vi "Test Copy from Pixmap Greyscale.vi"(8 "error in (no error)":errorcluster, 11 "Test Case In":refnum<class "Image.lvclass">) -> (0 "error out":errorcluster, 3 "Test Case Out":refnum<class "Image.lvclass">)   [LabVIEW 2020, in "test.lvlib" / "Image.lvclass"]
uses:
  Image.lvclass
  C:/Program Files (x86)/National Instruments/LabVIEW 2020/vi.lib/Astemes/LUnit/Test Case.lvclass
  <vilib>/picture/picture.llb/imagedata.ctl
  <vilib>/Astemes/LUnit/Test Case.lvclass/Test Case.ctl
  2c93f62b-78d7-4b59-b27c-14bd701a5d71.vi
  8166983f-db3b-480f-a786-a958408166cb.vi
  03fde0f0-e029-4dad-9f9a-a95d25ce423a.vi
  3bb2986f-6074-4300-8ef6-a7ee1c3ba308.vi
  02fb1d00-84d2-4392-bb0c-78c1f80e642d.vi
  image/New Image (Greyscale).vi
  image/Copy Pixmap to Image (Greyscale with Mask Output).vi
  image/Copy Pixmap to Image (Greyscale Flatten Mask).vi
  7f5bb767-9dbf-47d9-8f44-5f4901e96d00.vi
  e6d5ae8e-bd70-4c65-a769-b7cfb03e80c7.vi
  d454bffa-6717-48ab-b8d5-b1f03345aa55.vi
  image/New Image (Greyscale).vi/6598b9e0-8a08-46f5-91fd-ca1b87217137.vi
  image/Copy Pixmap to Image (Greyscale with Mask Output).vi/3b7a14f1-ed28-461e-8305-e3c68bcd5d6e.vi
  image/Copy Pixmap to Image (Greyscale Flatten Mask).vi/f0818824-bd55-4656-87f2-fcc208e7cf24.vi
  <vilib>/Astemes/LUnit/Append Pass Result.vi
  <vilib>/Astemes/LUnit/Append Fail Result.vi
  <vilib>/Astemes/LUnit/Describe Comparison.vi
  7f5bb767-9dbf-47d9-8f44-5f4901e96d00.vi/9c5d11cd-9439-4240-a1ee-d9baace9c924.vi
  e6d5ae8e-bd70-4c65-a769-b7cfb03e80c7.vi/9c5d11cd-9439-4240-a1ee-d9baace9c924.vi
  d454bffa-6717-48ab-b8d5-b1f03345aa55.vi/9c5d11cd-9439-4240-a1ee-d9baace9c924.vi
  image/FixPixmap.vi
  <vilib>/Astemes/LUnit/Run In UI.vi
  image/Default8bitColourMap.vi
  <vilib>/Utility/error.llb/Clear Errors.vi
  <vilib>/Utility/colorconv.llb/Color to RGB.vi
  common/Module Path.vi
  <vilib>/Utility/error.llb/Error Cluster From Error Code.vi
  <vilib>/Astemes/LUnit/Describe Variant.vi
  image/image.lvlib
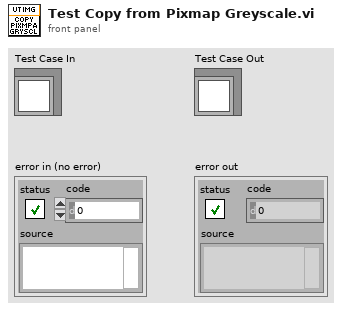
[diagram p1: front panel]
types:
  T1 = enum16{"8 Bit No Mask", "24 Bit No Mask", "32 Bit No Mask", "8 Bit Mask", "24 Bit Mask", "32 Bit Mask", "8 Pixels Wide Masked", "16 Pixels Wide Masked"}
  T2 = cluster{"left":i16, "top":i16, "right":i16, "bottom":i16}
  T3 = enum16{"8 Bit No Mask", "24 Bit No Mask", "32 Bit No Mask", "8 Bit Mask", "24 Bit Mask", "32 Bit Mask", "8 Pixels Wide Masked", "16 Pixels Wide Masked"}[]
  T4 = typedef "imagedata.ctl" = cluster{"image type":i32, "image depth":i32, "image":u8[], "mask":u8[], "colors":u32[], "Rectangle":cluster{"left":i16, "top":i16, "right":i16, "bottom":i16}}
  T5 = cluster{"8 No Mask":T4, "8 Mask":T4, "24 No Mask":T4, "24 Mask":T4, "32 No Mask":T4, "32 Mask":T4, "24 Mask - 8 wide":T4, "24 Mask - 16 wide":T4}
  T6 = typedef "image.lvlib/Greyscale Image.ctl" = refnum<data-value>
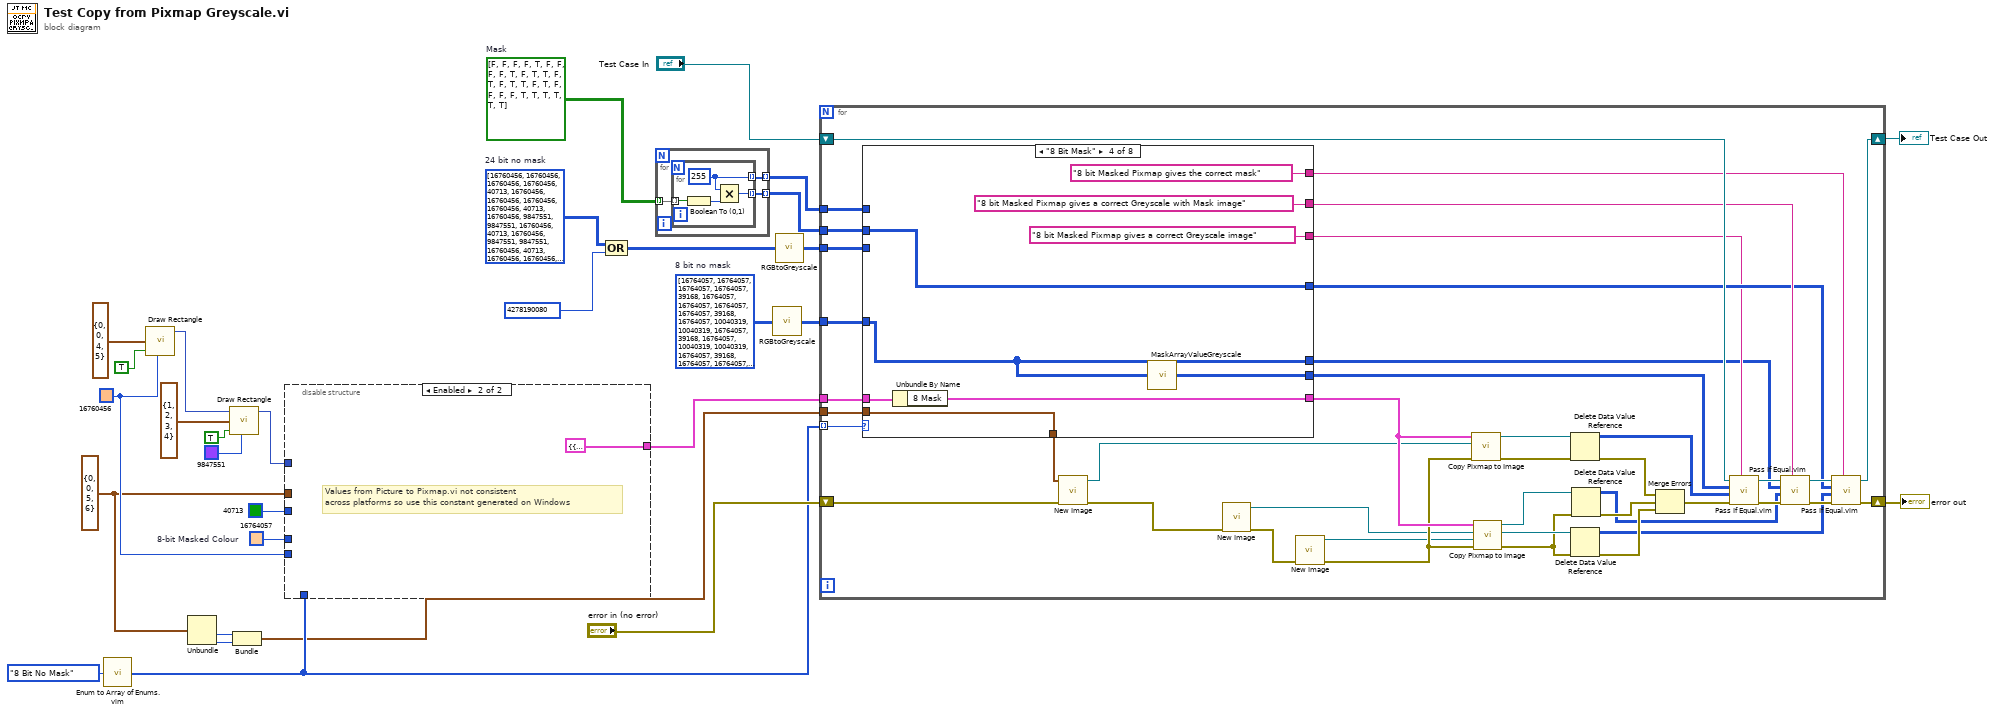
[diagram p0: block diagram]
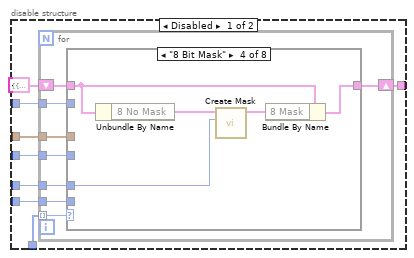
[diagram p2: hidden frame]
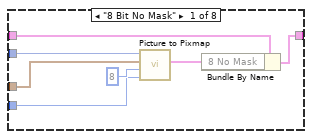
[diagram p3: hidden frame]
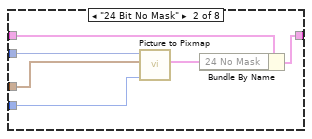
[diagram p4: hidden frame]
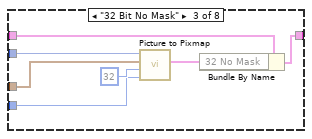
[diagram p5: hidden frame]
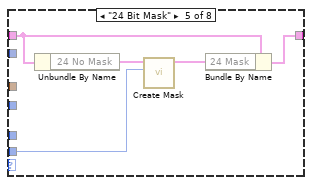
[diagram p6: hidden frame]
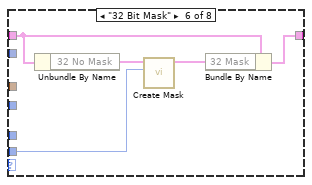
[diagram p7: hidden frame]
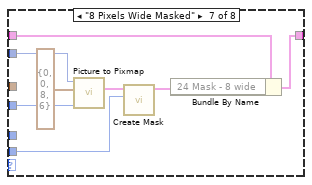
[diagram p8: hidden frame]
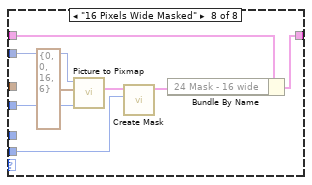
[diagram p9: hidden frame]
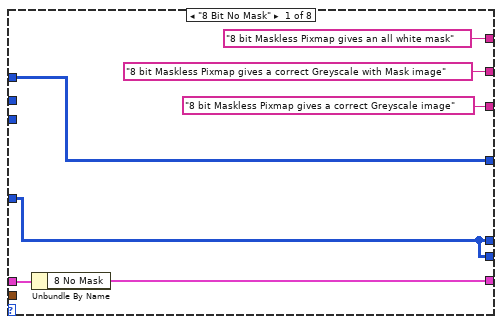
[diagram p10: hidden frame]
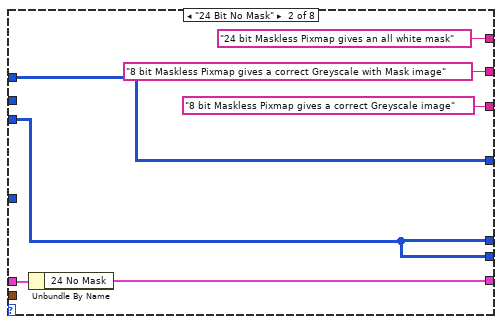
[diagram p11: hidden frame]
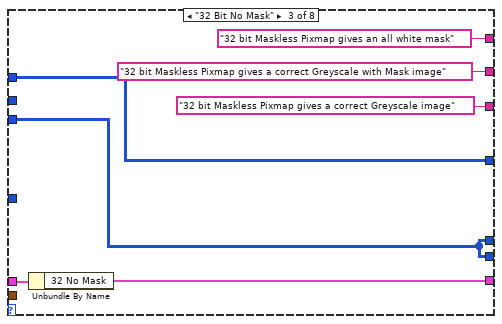
[diagram p12: hidden frame]
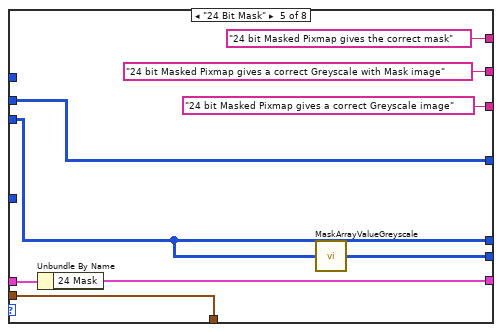
[diagram p13: hidden frame]
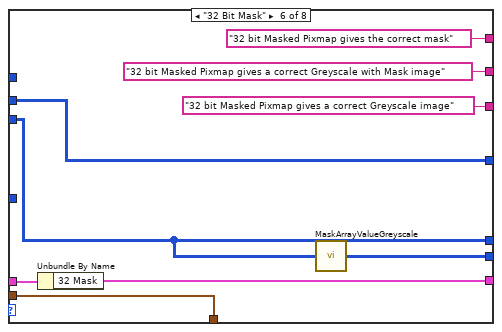
[diagram p14: hidden frame]
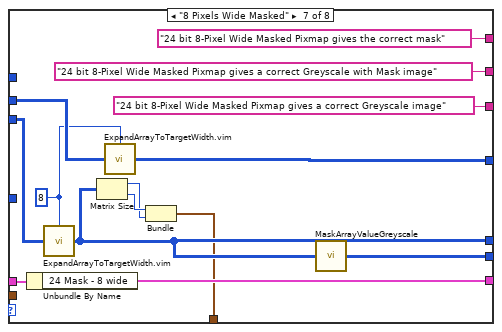
[diagram p15: hidden frame]
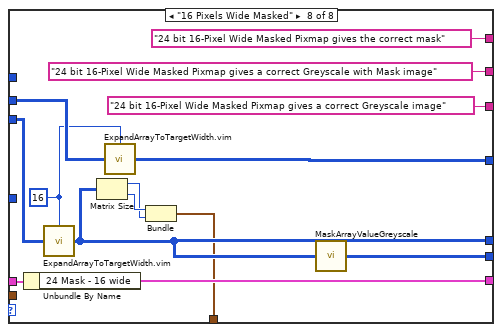
[diagram p16: hidden frame]
diagram:
  w5 = u32 16764057  # 8-bit Masked Colour
  w17 = bool[][] [[FALSE, FALSE, FALSE, FALSE, TRUE], [FALSE, FALSE, FALSE, FALSE, TRUE], [FALSE, TRUE, TRUE, FALSE, TRUE], [FALSE, TRUE, TRUE, FALSE, TRUE], [FALSE, FALSE, FALSE, FALSE, TRUE], [TRUE, TRUE, TRUE, TRUE, TRUE]]  # Mask
  w2 = u32[][] [[16764057, 16764057, 16764057, 16764057, 39168], [16764057, 16764057, 16764057, 16764057, 39168], [16764057, 10040319, 10040319, 16764057, 39168], [16764057, 10040319, 10040319, 16764057, 39168], [16764057, 16764057, 16764057, 16764057, 39168], [39168, 39168, 39168, 39168, 39168]]  # 8 bit no mask
  w20 = u32[][] [[16760456, 16760456, 16760456, 16760456, 40713], [16760456, 16760456, 16760456, 16760456, 40713], [16760456, 9847551, 9847551, 16760456, 40713], [16760456, 9847551, 9847551, 16760456, 40713], [16760456, 16760456, 16760456, 16760456, 40713], [40713, 40713, 40713, 40713, 40713]]  # 24 bit no mask
  w9 = T2 {"left"=0, "top"=0, "right"=5, "bottom"=6} ("rect")
  w12 = u32 16760456 ("color(black)")
  n1 = call "Enum to Array of Enums.vim"("enum"=T1."8 Bit No Mask") -> ("array of enums"=w15:T3)
  n2 = call <vilib>:"Draw Rectangle.vi"("rect"=T2 {"left"=0, "top"=0, "right"=4, "bottom"=5}, "fill?(F)"=TRUE, "color(black)"=w12) -> ("new picture"=w30:picture)  [unwired: 6 in]
  n3 = Unbundle(w9) -> ("right"=w8:i16, "bottom"=w7:i16)  [unwired: 2 out]
  n4 = call <vilib>:"Draw Rectangle.vi"("picture"=w30, "rect"=T2 {"left"=1, "top"=2, "right"=3, "bottom"=4}, "fill?(F)"=TRUE, "color(black)"=u32 9847551) -> ("new picture"=w13:picture)  [unwired: 5 in]
  n5 = Bundle("right"=w8, "bottom"=w7) -> (w6:cluster{"right":i16, "bottom":i16})  [unwired: 1 in]
  n6 = disable-structure shown="Enabled" {
    disable-tunnel: w15 -> [w38 _]
    disable-tunnel: [w36 T5 {"8 No Mask"={"image type"=0, "image depth"=8, "image"=[8, 8, 8, 8, 197, 0, 8, 8, 8, 8, 197, 0, 8, 96, 96, 8, 197, 0, 8, 96, 96, 8, 197, 0, 8, 8, 8, 8, 197, 0, 197, 197, 197, 197, 197, 0], "mask"=[], "colors"=[16777215, 16777164, 16777113, 16777062, 16777011, 16776960, 16764159, 16764108, 16764057, 16764006, 16763955, 16763904, 16751103, 16751052, 16751001, 16750950, 16750899, 16750848, 16738047, 16737996, 16737945, 16737894, 16737843, 16737792, 16724991, 16724940, 16724889, 16724838, 16724787, 16724736, 16711935, 16711884, 16711833, 16711782, 16711731, 16711680, 13434879, 13434828, 13434777, 13434726, 13434675, 13434624, 13421823, 13421772, 13421721, 13421670, 13421619, 13421568, 13408767, 13408716, 13408665, 13408614, 13408563, 13408512, 13395711, 13395660, 13395609, 13395558, 13395507, 13395456, 13382655, 13382604, 13382553, 13382502, 13382451, 13382400, 13369599, 13369548, 13369497, 13369446, 13369395, 13369344, 10092543, 10092492, 10092441, 10092390, 10092339, 10092288, 10079487, 10079436, 10079385, 10079334, 10079283, 10079232, 10066431, 10066380, 10066329, 10066278, 10066227, 10066176, 10053375, 10053324, 10053273, 10053222, 10053171, 10053120, 10040319, 10040268, 10040217, 10040166, 10040115, 10040064, 10027263, 10027212, 10027161, 10027110, 10027059, 10027008, 6750207, 6750156, 6750105, 6750054, 6750003, 6749952, 6737151, 6737100, 6737049, 6736998, 6736947, 6736896, 6724095, 6724044, 6723993, 6723942, 6723891, 6723840, 6711039, 6710988, 6710937, 6710886, 6710835, 6710784, 6697983, 6697932, 6697881, 6697830, 6697779, 6697728, 6684927, 6684876, 6684825, 6684774, 6684723, 6684672, 3407871, 3407820, 3407769, 3407718, 3407667, 3407616, 3394815, 3394764, 3394713, 3394662, 3394611, 3394560, 3381759, 3381708, 3381657, 3381606, 3381555, 3381504, 3368703, 3368652, 3368601, 3368550, 3368499, 3368448, 3355647, 3355596, 3355545, 3355494, 3355443, 3355392, 3342591, 3342540, 3342489, 3342438, 3342387, 3342336, 65535, 65484, 65433, 65382, 65331, 65280, 52479, 52428, 52377, 52326, 52275, 52224, 39423, 39372, 39321, 39270, 39219, 39168, 26367, 26316, 26265, 26214, 26163, 26112, 13311, 13260, 13209, 13158, 13107, 13056, 255, 204, 153, 102, 51, 15597568, 14483456, 12255232, 11141120, 8912896, 7798784, 5570560, 4456448, 2228224, 1114112, 60928, 56576, 47872, 43520, 34816, 30464, 21760, 17408, 8704, 4352, 238, 221, 187, 170, 136, 119, 85, 68, 34, 17, 15658734, 14540253, 12303291, 11184810, 8947848, 7829367, 5592405, 4473924, 2236962, 1118481, 0], "Rectangle"={"left"=0, "top"=0, "right"=5, "bottom"=6}}, "8 Mask"={"image type"=0, "image depth"=8, "image"=[8, 8, 8, 8, 197, 0, 8, 8, 8, 8, 197, 0, 8, 96, 96, 8, 197, 0, 8, 96, 96, 8, 197, 0, 8, 8, 8, 8, 197, 0, 197, 197, 197, 197, 197, 0], "mask"=[15, 255, 15, 255, 111, 255, 111, 255, 15, 255, 255, 255], "colors"=[16777215, 16777164, 16777113, 16777062, 16777011, 16776960, 16764159, 16764108, 16764057, 16764006, 16763955, 16763904, 16751103, 16751052, 16751001, 16750950, 16750899, 16750848, 16738047, 16737996, 16737945, 16737894, 16737843, 16737792, 16724991, 16724940, 16724889, 16724838, 16724787, 16724736, 16711935, 16711884, 16711833, 16711782, 16711731, 16711680, 13434879, 13434828, 13434777, 13434726, 13434675, 13434624, 13421823, 13421772, 13421721, 13421670, 13421619, 13421568, 13408767, 13408716, 13408665, 13408614, 13408563, 13408512, 13395711, 13395660, 13395609, 13395558, 13395507, 13395456, 13382655, 13382604, 13382553, 13382502, 13382451, 13382400, 13369599, 13369548, 13369497, 13369446, 13369395, 13369344, 10092543, 10092492, 10092441, 10092390, 10092339, 10092288, 10079487, 10079436, 10079385, 10079334, 10079283, 10079232, 10066431, 10066380, 10066329, 10066278, 10066227, 10066176, 10053375, 10053324, 10053273, 10053222, 10053171, 10053120, 10040319, 10040268, 10040217, 10040166, 10040115, 10040064, 10027263, 10027212, 10027161, 10027110, 10027059, 10027008, 6750207, 6750156, 6750105, 6750054, 6750003, 6749952, 6737151, 6737100, 6737049, 6736998, 6736947, 6736896, 6724095, 6724044, 6723993, 6723942, 6723891, 6723840, 6711039, 6710988, 6710937, 6710886, 6710835, 6710784, 6697983, 6697932, 6697881, 6697830, 6697779, 6697728, 6684927, 6684876, 6684825, 6684774, 6684723, 6684672, 3407871, 3407820, 3407769, 3407718, 3407667, 3407616, 3394815, 3394764, 3394713, 3394662, 3394611, 3394560, 3381759, 3381708, 3381657, 3381606, 3381555, 3381504, 3368703, 3368652, 3368601, 3368550, 3368499, 3368448, 3355647, 3355596, 3355545, 3355494, 3355443, 3355392, 3342591, 3342540, 3342489, 3342438, 3342387, 3342336, 65535, 65484, 65433, 65382, 65331, 65280, 52479, 52428, 52377, 52326, 52275, 52224, 39423, 39372, 39321, 39270, 39219, 39168, 26367, 26316, 26265, 26214, 26163, 26112, 13311, 13260, 13209, 13158, 13107, 13056, 255, 204, 153, 102, 51, 15597568, 14483456, 12255232, 11141120, 8912896, 7798784, 5570560, 4456448, 2228224, 1114112, 60928, 56576, 47872, 43520, 34816, 30464, 21760, 17408, 8704, 4352, 238, 221, 187, 170, 136, 119, 85, 68, 34, 17, 15658734, 14540253, 12303291, 11184810, 8947848, 7829367, 5592405, 4473924, 2236962, 1118481, 0], "Rectangle"={"left"=0, "top"=0, "right"=5, "bottom"=6}}, "24 No Mask"={"image type"=0, "image depth"=24, "image"=[255, 190, 136, 255, 190, 136, 255, 190, 136, 255, 190, 136, 0, 159, 9, 255, 190, 136, 255, 190, 136, 255, 190, 136, 255, 190, 136, 0, 159, 9, 255, 190, 136, 150, 66, 255, 150, 66, 255, 255, 190, 136, 0, 159, 9, 255, 190, 136, 150, 66, 255, 150, 66, 255, 255, 190, 136, 0, 159, 9, 255, 190, 136, 255, 190, 136, 255, 190, 136, 255, 190, 136, 0, 159, 9, 0, 159, 9, 0, 159, 9, 0, 159, 9, 0, 159, 9, 0, 159, 9], "mask"=[], "colors"=[], "Rectangle"={"left"=0, "top"=0, "right"=5, "bottom"=6}}, "24 Mask"={"image type"=0, "image depth"=24, "image"=[255, 190, 136, 255, 190, 136, 255, 190, 136, 255, 190, 136, 0, 159, 9, 255, 190, 136, 255, 190, 136, 255, 190, 136, 255, 190, 136, 0, 159, 9, 255, 190, 136, 150, 66, 255, 150, 66, 255, 255, 190, 136, 0, 159, 9, 255, 190, 136, 150, 66, 255, 150, 66, 255, 255, 190, 136, 0, 159, 9, 255, 190, 136, 255, 190, 136, 255, 190, 136, 255, 190, 136, 0, 159, 9, 0, 159, 9, 0, 159, 9, 0, 159, 9, 0, 159, 9, 0, 159, 9], "mask"=[15, 255, 15, 255, 111, 255, 111, 255, 15, 255, 255, 255], "colors"=[], "Rectangle"={"left"=0, "top"=0, "right"=5, "bottom"=6}}, "32 No Mask"={"image type"=0, "image depth"=24, "image"=[255, 190, 136, 255, 190, 136, 255, 190, 136, 255, 190, 136, 0, 159, 9, 255, 190, 136, 255, 190, 136, 255, 190, 136, 255, 190, 136, 0, 159, 9, 255, 190, 136, 150, 66, 255, 150, 66, 255, 255, 190, 136, 0, 159, 9, 255, 190, 136, 150, 66, 255, 150, 66, 255, 255, 190, 136, 0, 159, 9, 255, 190, 136, 255, 190, 136, 255, 190, 136, 255, 190, 136, 0, 159, 9, 0, 159, 9, 0, 159, 9, 0, 159, 9, 0, 159, 9, 0, 159, 9], "mask"=[], "colors"=[], "Rectangle"={"left"=0, "top"=0, "right"=5, "bottom"=6}}, "32 Mask"={"image type"=0, "image depth"=24, "image"=[255, 190, 136, 255, 190, 136, 255, 190, 136, 255, 190, 136, 0, 159, 9, 255, 190, 136, 255, 190, 136, 255, 190, 136, 255, 190, 136, 0, 159, 9, 255, 190, 136, 150, 66, 255, 150, 66, 255, 255, 190, 136, 0, 159, 9, 255, 190, 136, 150, 66, 255, 150, 66, 255, 255, 190, 136, 0, 159, 9, 255, 190, 136, 255, 190, 136, 255, 190, 136, 255, 190, 136, 0, 159, 9, 0, 159, 9, 0, 159, 9, 0, 159, 9, 0, 159, 9, 0, 159, 9], "mask"=[15, 255, 15, 255, 111, 255, 111, 255, 15, 255, 255, 255], "colors"=[], "Rectangle"={"left"=0, "top"=0, "right"=5, "bottom"=6}}, "24 Mask - 8 wide"={"image type"=0, "image depth"=24, "image"=[255, 190, 136, 255, 190, 136, 255, 190, 136, 255, 190, 136, 0, 159, 9, 0, 159, 9, 0, 159, 9, 0, 159, 9, 255, 190, 136, 255, 190, 136, 255, 190, 136, 255, 190, 136, 0, 159, 9, 0, 159, 9, 0, 159, 9, 0, 159, 9, 255, 190, 136, 150, 66, 255, 150, 66, 255, 255, 190, 136, 0, 159, 9, 0, 159, 9, 0, 159, 9, 0, 159, 9, 255, 190, 136, 150, 66, 255, 150, 66, 255, 255, 190, 136, 0, 159, 9, 0, 159, 9, 0, 159, 9, 0, 159, 9, 255, 190, 136, 255, 190, 136, 255, 190, 136, 255, 190, 136, 0, 159, 9, 0, 159, 9, 0, 159, 9, 0, 159, 9, 0, 159, 9, 0, 159, 9, 0, 159, 9, 0, 159, 9, 0, 159, 9, 0, 159, 9, 0, 159, 9, 0, 159, 9], "mask"=[15, 255, 15, 255, 111, 255, 111, 255, 15, 255, 255, 255], "colors"=[], "Rectangle"={"left"=0, "top"=0, "right"=8, "bottom"=6}}, "24 Mask - 16 wide"={"image type"=0, "image depth"=24, "image"=[255, 190, 136, 255, 190, 136, 255, 190, 136, 255, 190, 136, 0, 159, 9, 0, 159, 9, 0, 159, 9, 0, 159, 9, 0, 159, 9, 0, 159, 9, 0, 159, 9, 0, 159, 9, 0, 159, 9, 0, 159, 9, 0, 159, 9, 0, 159, 9, 255, 190, 136, 255, 190, 136, 255, 190, 136, 255, 190, 136, 0, 159, 9, 0, 159, 9, 0, 159, 9, 0, 159, 9, 0, 159, 9, 0, 159, 9, 0, 159, 9, 0, 159, 9, 0, 159, 9, 0, 159, 9, 0, 159, 9, 0, 159, 9, 255, 190, 136, 150, 66, 255, 150, 66, 255, 255, 190, 136, 0, 159, 9, 0, 159, 9, 0, 159, 9, 0, 159, 9, 0, 159, 9, 0, 159, 9, 0, 159, 9, 0, 159, 9, 0, 159, 9, 0, 159, 9, 0, 159, 9, 0, 159, 9, 255, 190, 136, 150, 66, 255, 150, 66, 255, 255, 190, 136, 0, 159, 9, 0, 159, 9, 0, 159, 9, 0, 159, 9, 0, 159, 9, 0, 159, 9, 0, 159, 9, 0, 159, 9, 0, 159, 9, 0, 159, 9, 0, 159, 9, 0, 159, 9, 255, 190, 136, 255, 190, 136, 255, 190, 136, 255, 190, 136, 0, 159, 9, 0, 159, 9, 0, 159, 9, 0, 159, 9, 0, 159, 9, 0, 159, 9, 0, 159, 9, 0, 159, 9, 0, 159, 9, 0, 159, 9, 0, 159, 9, 0, 159, 9, 0, 159, 9, 0, 159, 9, 0, 159, 9, 0, 159, 9, 0, 159, 9, 0, 159, 9, 0, 159, 9, 0, 159, 9, 0, 159, 9, 0, 159, 9, 0, 159, 9, 0, 159, 9, 0, 159, 9, 0, 159, 9, 0, 159, 9, 0, 159, 9], "mask"=[15, 255, 15, 255, 111, 255, 111, 255, 15, 255, 255, 255], "colors"=[], "Rectangle"={"left"=0, "top"=0, "right"=16, "bottom"=6}}} ("output cluster")] -> w14
    disable-tunnel: w13 -> [w35 _]
    disable-tunnel: w12 -> [w34 _]
    disable-tunnel: u32 40713 ("Background Color") -> [w33 _]
    disable-tunnel: w9 -> [w32 _]
    disable-tunnel: w5 -> [w31 _]
    frame Disabled {
      n7 = for {
        tunnel: w38 -> [w44] mode=indexing
        shift-right: [w45] -> w36
        shift-left: T5 {"8 No Mask"={"image type"=0, "image depth"=0, "image"=[], "mask"=[], "colors"=[], "Rectangle"={"left"=0, "top"=0, "right"=0, "bottom"=0}}, "8 Mask"={"image type"=0, "image depth"=0, "image"=[], "mask"=[], "colors"=[], "Rectangle"={"left"=0, "top"=0, "right"=0, "bottom"=0}}, "24 No Mask"={"image type"=0, "image depth"=0, "image"=[], "mask"=[], "colors"=[], "Rectangle"={"left"=0, "top"=0, "right"=0, "bottom"=0}}, "24 Mask"={"image type"=0, "image depth"=0, "image"=[], "mask"=[], "colors"=[], "Rectangle"={"left"=0, "top"=0, "right"=0, "bottom"=0}}, "32 No Mask"={"image type"=0, "image depth"=0, "image"=[], "mask"=[], "colors"=[], "Rectangle"={"left"=0, "top"=0, "right"=0, "bottom"=0}}, "32 Mask"={"image type"=0, "image depth"=0, "image"=[], "mask"=[], "colors"=[], "Rectangle"={"left"=0, "top"=0, "right"=0, "bottom"=0}}, "24 Mask - 8 wide"={"image type"=0, "image depth"=0, "image"=[], "mask"=[], "colors"=[], "Rectangle"={"left"=0, "top"=0, "right"=0, "bottom"=0}}, "24 Mask - 16 wide"={"image type"=0, "image depth"=0, "image"=[], "mask"=[], "colors"=[], "Rectangle"={"left"=0, "top"=0, "right"=0, "bottom"=0}}} ("output cluster") -> [w46]
        tunnel: w35 -> [w42]
        tunnel: w32 -> [w43]
        tunnel: w33 -> [w41]
        tunnel: w34 -> [w40]
        tunnel: w31 -> [w39]
        n8 = case shown="\"8 Bit Mask\"" w44 {
          tunnel: w46 -> [w53 w59 w66 w70 w75 w80 w89 w97]
          tunnel: [w52 w58 w65 w71 w76 w81 w88 w96] -> w45
          tunnel: w43 -> [w50 w57 w63 _ _ _ _ _]
          tunnel: w42 -> [w49 w56 w62 _ _ _ w85 w93]
          tunnel: w41 -> [w47 w54 w60 _ _ _ w84 w92]
          tunnel: w40 -> [_ _ _ _ w72 w77 w82 w90]
          tunnel: w39 -> [_ _ _ w67 _ _ _ _]
          frame "8 Bit No Mask" {
            n9 = call <vilib>:"Picture to Pixmap.vi"("Background Color"=w47, "depth"=8, "rect"=w50, "picture"=w49) -> ("image data"=w48:T4)  [unwired: 6 in, 1 out]
            n10 = Bundle By Name(cluster=w53, "8 No Mask"=w48) -> (w52:T5)
          }
          frame "24 Bit No Mask" {
            n11 = call <vilib>:"Picture to Pixmap.vi"("Background Color"=w54, "rect"=w57, "picture"=w56) -> ("image data"=w55:T4)  [unwired: 7 in, 1 out]
            n12 = Bundle By Name(cluster=w59, "24 No Mask"=w55) -> (w58:T5)
          }
          frame "32 Bit No Mask" {
            n13 = call <vilib>:"Picture to Pixmap.vi"("Background Color"=w60, "depth"=32, "rect"=w63, "picture"=w62) -> ("image data"=w61:T4)  [unwired: 6 in, 1 out]
            n14 = Bundle By Name(cluster=w66, "32 No Mask"=w61) -> (w65:T5)
          }
          frame "8 Bit Mask" {
            n15 = Unbundle By Name(w70) -> ("8 No Mask"=w69:T4)
            n16 = call <vilib>:"Create Mask.vi"("Mask Color (Black)"=w67, "image data"=w69) -> ("image data"=w68:T4)  [unwired: 9 in]
            n17 = Bundle By Name(cluster=w70, "8 Mask"=w68) -> (w71:T5)
          }
          frame "24 Bit Mask" {
            n18 = Unbundle By Name(w75) -> ("24 No Mask"=w74:T4)
            n19 = call <vilib>:"Create Mask.vi"("Mask Color (Black)"=w72, "image data"=w74) -> ("image data"=w73:T4)  [unwired: 9 in]
            n20 = Bundle By Name(cluster=w75, "24 Mask"=w73) -> (w76:T5)
          }
          frame "32 Bit Mask" {
            n21 = Unbundle By Name(w80) -> ("32 No Mask"=w79:T4)
            n22 = call <vilib>:"Create Mask.vi"("Mask Color (Black)"=w77, "image data"=w79) -> ("image data"=w78:T4)  [unwired: 9 in]
            n23 = Bundle By Name(cluster=w80, "32 Mask"=w78) -> (w81:T5)
          }
          frame "8 Pixels Wide Masked" {
            n24 = call <vilib>:"Picture to Pixmap.vi"("Background Color"=w84, "rect"=T2 {"left"=0, "top"=0, "right"=8, "bottom"=6}, "picture"=w85) -> ("image data"=w87:T4)  [unwired: 7 in, 1 out]
            n25 = call <vilib>:"Create Mask.vi"("Mask Color (Black)"=w82, "image data"=w87) -> ("image data"=w86:T4)  [unwired: 9 in]
            n26 = Bundle By Name(cluster=w89, "24 Mask - 8 wide"=w86) -> (w88:T5)
          }
          frame "16 Pixels Wide Masked" {
            n27 = call <vilib>:"Picture to Pixmap.vi"("Background Color"=w92, "rect"=T2 {"left"=0, "top"=0, "right"=16, "bottom"=6}, "picture"=w93) -> ("image data"=w95:T4)  [unwired: 7 in, 1 out]
            n28 = call <vilib>:"Create Mask.vi"("Mask Color (Black)"=w90, "image data"=w95) -> ("image data"=w94:T4)  [unwired: 9 in]
            n29 = Bundle By Name(cluster=w97, "24 Mask - 16 wide"=w94) -> (w96:T5)
          }
        }
      }
    }
    frame Enabled {
      # "Values from Picture to Pixmap.vi not consistent\nacross platforms so use this constant generated on Windows"
    }
  }
  n30 = Compound Arithmetic op=OR(w20, u32 4278190080) -> (w19:u32[][])
  n31 = for "Masks" {
    tunnel: w17 -> [w100] mode=indexing
    tunnel: [w101] -> w18 mode=indexing
    tunnel: [w99] -> w16 mode=indexing
    n32 = for {
      tunnel: [w104] -> w101 mode=indexing
      tunnel: w100 -> [w105] mode=indexing
      tunnel: [w103] -> w99 mode=indexing
      w104 = u8 255 ("unsigned 8bit integer")
      n33 = Boolean To (0,1)(Boolean=w105) -> (0, 1=w102:i16)
      n34 = Multiply(x=w104, y=w102) -> (x*y=w103:u8)
    }
  }
  n35 = call "RGBtoGreyscale.vi"("RBG"=w2) -> ("Greyscale"=w3:u8[][])
  n36 = call "RGBtoGreyscale.vi"("RBG"=w19) -> ("Greyscale"=w1:u8[][])
  n37 = for {
    tunnel: w14 -> [w146]
    tunnel: w15 -> [w140] mode=indexing
    shift-right: [w131] -> w21
    shift-left: "error in (no error)" -> [w123]
    shift-right: [w130] -> w24
    shift-left: "Test Case In" -> [w139]
    tunnel: w1 -> [w124]
    tunnel: w3 -> [w127]
    tunnel: w18 -> [w120]
    tunnel: w16 -> [w119]
    tunnel: w6 -> [w114]
    n38 = case shown="\"8 Bit Mask\"" w140 {
      tunnel: w146 -> [w153 w160 w167 w176 w185 w194 w208 w222]
      tunnel: [w152 w159 w166 w175 w184 w193 w207 w221] -> w145
      tunnel: ["8 bit Maskless Pixmap gives an all white mask" ("Description") "24 bit Maskless Pixmap gives an all white mask" ("Description") "32 bit Maskless Pixmap gives an all white mask" ("Description") "8 bit Masked Pixmap gives the correct mask" ("Description") "24 bit Masked Pixmap gives the correct mask" ("Description") "32 bit Masked Pixmap gives the correct mask" ("Description") "24 bit 8-Pixel Wide Masked Pixmap gives the correct mask" ("Description") "24 bit 16-Pixel Wide Masked Pixmap gives the correct mask" ("Description")] -> w129
      tunnel: ["8 bit Maskless Pixmap gives a correct Greyscale with Mask image" ("Description") "8 bit Maskless Pixmap gives a correct Greyscale with Mask image" ("Description") "32 bit Maskless Pixmap gives a correct Greyscale with Mask image" ("Description") "8 bit Masked Pixmap gives a correct Greyscale with Mask image" ("Description") "24 bit Masked Pixmap gives a correct Greyscale with Mask image" ("Description") "32 bit Masked Pixmap gives a correct Greyscale with Mask image" ("Description") "24 bit 8-Pixel Wide Masked Pixmap gives a correct Greyscale with Mask image" ("Description") "24 bit 16-Pixel Wide Masked Pixmap gives a correct Greyscale with Mask image" ("Description")] -> w128
      tunnel: [w149 w154 w161 w169 w179 w188 w203 w217] -> w107
      tunnel: w127 -> [w149 _ _ w172 _ _ _ _]
      tunnel: [w149 w154 w161 w172 w177 w186 w198 w212] -> w108
      tunnel: [w147 w155 w162 w168 w178 w187 w200 w214] -> w126
      tunnel: ["8 bit Maskless Pixmap gives a correct Greyscale image" ("Description") "8 bit Maskless Pixmap gives a correct Greyscale image" ("Description") "32 bit Maskless Pixmap gives a correct Greyscale image" ("Description") "8 bit Masked Pixmap gives a correct Greyscale image" ("Description") "24 bit Masked Pixmap gives a correct Greyscale image" ("Description") "32 bit Masked Pixmap gives a correct Greyscale image" ("Description") "24 bit 8-Pixel Wide Masked Pixmap gives a correct Greyscale image" ("Description") "24 bit 16-Pixel Wide Masked Pixmap gives a correct Greyscale image" ("Description")] -> w125
      tunnel: w124 -> [_ w154 w161 _ w177 w186 w201 w215]
      tunnel: w120 -> [w147 w155 w162 _ _ _ _ _]
      tunnel: w119 -> [_ _ _ w168 w178 w187 w202 w216]
      tunnel: [_ _ _ w170 w180 w189 w195 w209] -> w115
      tunnel: w114 -> [_ _ _ w170 w180 w189 _ _]
      frame "8 Bit No Mask" {
        n39 = Unbundle By Name(w153) -> ("8 No Mask"=w152:T4)
      }
      frame "24 Bit No Mask" {
        n40 = Unbundle By Name(w160) -> ("24 No Mask"=w159:T4)
      }
      frame "32 Bit No Mask" {
        n41 = Unbundle By Name(w167) -> ("32 No Mask"=w166:T4)
      }
      frame "8 Bit Mask" {
        n42 = Unbundle By Name(w176) -> ("8 Mask"=w175:T4)
        n43 = call "MaskArrayValueGreyscale.vi"("Array In"=w172) -> ("Array out"=w169:u8[][])
      }
      frame "24 Bit Mask" {
        n44 = Unbundle By Name(w185) -> ("24 Mask"=w184:T4)
        n45 = call "MaskArrayValueGreyscale.vi"("Array In"=w177) -> ("Array out"=w179:u8[][])
      }
      frame "32 Bit Mask" {
        n46 = Unbundle By Name(w194) -> ("32 Mask"=w193:T4)
        n47 = call "MaskArrayValueGreyscale.vi"("Array In"=w186) -> ("Array out"=w188:u8[][])
      }
      frame "8 Pixels Wide Masked" {
        w199 = 8 ("Target Width")
        n48 = Unbundle By Name(w208) -> ("24 Mask - 8 wide"=w207:T4)
        n49 = call "ExpandArrayToTargetWidth.vim"("Array in"=w201, "Target Width"=w199) -> ("Array out"=w198:u8[][])
        n50 = Matrix Size(0:w198) -> (1:w196:i32, 2:w197:i32)
        n51 = call "ExpandArrayToTargetWidth.vim"("Array in"=w202, "Target Width"=w199) -> ("Array out"=w200:u8[][])
        n52 = Bundle("matrix"=w197, "number of columns"=w196) -> (w195:cluster{"matrix":i32, "number of columns":i32})  [unwired: 1 in]
        n53 = call "MaskArrayValueGreyscale.vi"("Array In"=w198) -> ("Array out"=w203:u8[][])
      }
      frame "16 Pixels Wide Masked" {
        w213 = 16 ("Target Width")
        n54 = Unbundle By Name(w222) -> ("24 Mask - 16 wide"=w221:T4)
        n55 = call "ExpandArrayToTargetWidth.vim"("Array in"=w215, "Target Width"=w213) -> ("Array out"=w212:u8[][])
        n56 = Matrix Size(0:w212) -> (1:w210:i32, 2:w211:i32)
        n57 = call "ExpandArrayToTargetWidth.vim"("Array in"=w216, "Target Width"=w213) -> ("Array out"=w214:u8[][])
        n58 = Bundle("matrix"=w211, "number of columns"=w210) -> (w209:cluster{"matrix":i32, "number of columns":i32})  [unwired: 1 in]
        n59 = call "MaskArrayValueGreyscale.vi"("Array In"=w212) -> ("Array out"=w217:u8[][])
      }
    }
    n60 = call-poly "New Image.vi"("error in (no error)"=w123, "Preallocated Image Size (Default 0,0)"=w115) -> ("error out"=w122:errorcluster, "New Greyscale Image"=w121:T6)  [unwired: 8 in]
    n61 = call-poly "New Image.vi"("error in (no error)"=w122) -> ("error out"=w118:errorcluster, "New Greyscale Image"=w116:T6)  [unwired: 9 in]
    n62 = call-poly "New Image.vi"("error in (no error)"=w118) -> ("error out"=w144:errorcluster, "New Greyscale Image"=w117:T6)  [unwired: 9 in]
    n63 = call-poly "Copy Pixmap to Image.vi"("error in (no error)"=w144, "Greyscale Image Destination"=w121, "Pixmap Image Data"=w145) -> ("error out"=w110:errorcluster, "Greyscale Image Destination (duplicate)"=w109:T6)  [unwired: 7 in]
    n64 = call-poly "Copy Pixmap to Image.vi"("error in (no error)"=w144, "Greyscale Image Mask"=w117, "Greyscale Image Destination"=w116, "Pixmap Image Data"=w145) -> ("error out"=w112:errorcluster, "Greyscale Image Mask (duplicate)"=w113:T6, "Greyscale Image Destination (duplicate)"=w111:T6)  [unwired: 5 in]
    n65 = Delete Data Value Reference(data value reference=w109, error in=w110) -> (data value=w106:u8[][], error out=w143:errorcluster)
    n66 = Delete Data Value Reference(data value reference=w113, error in=w112) -> (data value=w133:u8[][], error out=w141:errorcluster)
    n67 = Delete Data Value Reference(data value reference=w111, error in=w112) -> (data value=w134:u8[][], error out=w142:errorcluster)
    n68 = Merge Errors(w143, w142, w141) -> (w132:errorcluster)
    n69 = call "Pass If Equal.vim"("Description"=w125, "error in (no error)"=w132, "Actual"=w106, "Expected"=w107, "LUnit Test Case In"=w139) -> ("error out"=w136:errorcluster, "LUnit Test Case Out"=w138:refnum<class "Image.lvclass">)  [unwired: 5 in]
    n70 = call "Pass If Equal.vim"("Description"=w128, "error in (no error)"=w136, "Actual"=w134, "Expected"=w108, "LUnit Test Case In"=w138) -> ("error out"=w135:errorcluster, "LUnit Test Case Out"=w137:refnum<class "Image.lvclass">)  [unwired: 5 in]
    n71 = call "Pass If Equal.vim"("Description"=w129, "error in (no error)"=w135, "Actual"=w133, "Expected"=w126, "LUnit Test Case In"=w137) -> ("error out"=w131:errorcluster, "LUnit Test Case Out"=w130:refnum<class "Image.lvclass">)  [unwired: 5 in]
  }
  "error out" <- w21
  "Test Case Out" <- w24
